vi "未命名 3.vi"() -> ()   [LabVIEW 2019]
panel:
  out "波形图表":T1(graph)
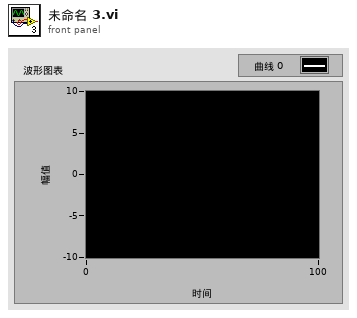
[diagram p1: front panel]
types:
  T1 = cluster{"number: 0 to 1":dbl, "number: 0 to 1":dbl}
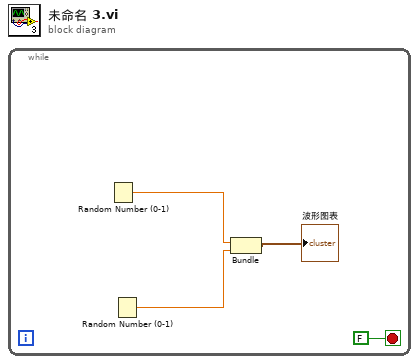
[diagram p0: block diagram]
diagram:
  n1 = while {
    stop <- FALSE stop-if-true
    n2 = Random Number (0-1)() -> (number: 0 to 1=w4:dbl)
    n3 = Random Number (0-1)() -> (number: 0 to 1=w3:dbl)
    n4 = Bundle("number: 0 to 1"=w4, "number: 0 to 1"=w3) -> (→"波形图表":T1)  [unwired: 1 in]
  }
